vi "例4-27.vi"() -> ()   [LabVIEW 2019]
panel:
  out "波形图":cluster{dbl[]}[](graph)
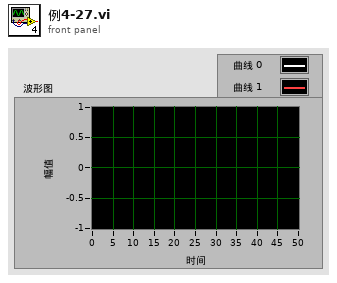
[diagram p1: front panel]
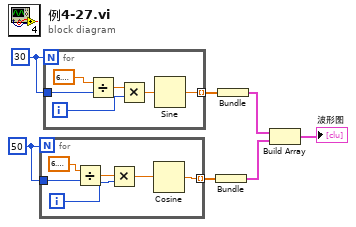
[diagram p0: block diagram]
diagram:
  w6 = 50
  w7 = 30
  n1 = for {
    N: w6 -> [_]
    tunnel: w6 -> [w11]
    tunnel: [w8] -> w4 mode=indexing
    i -> [w10]
    n2 = Divide(x=6.283185307179586, y=w11) -> (x/y=w13:dbl)
    n3 = Multiply(x=w13, y=w10) -> (x*y=w9:dbl)
    n4 = Cosine(x=w9) -> (cos(x)=w8:dbl)
  }
  n5 = for {
    N: w7 -> [_]
    tunnel: w7 -> [w16]
    tunnel: [w14] -> w5 mode=indexing
    i -> [w15]
    n6 = Divide(x=6.283185307179586, y=w16) -> (x/y=w18:dbl)
    n7 = Multiply(x=w18, y=w15) -> (x*y=w17:dbl)
    n8 = Sine(x=w17) -> (sin(x)=w14:dbl)
  }
  n9 = Bundle(w4) -> (w2:cluster{dbl[]})  [unwired: 1 in]
  n10 = Bundle(w5) -> (w3:cluster{dbl[]})  [unwired: 1 in]
  n11 = Build Array(w3, w2) -> (→"波形图":cluster{dbl[]}[])
